vi "Test Read Speed.vi"(8 "error in (no error)":errorcluster, 11 "Path":path) -> (0 "error out":errorcluster, 2 "Read Times":T1)   [LabVIEW 2016]
uses:
  Data/Typedefs/Dictionary--cluster.ctl
  Data/Data.lvclass
  <vilib>/Utility/Data Type/NI_Data Type.lvlib
panel:
  out "Data (Dictionary)":T2[](array[typedef])=[{"key"="time", "value"=variant(dbl[] array[87118 elements])}, {"key"="temp", "value"=variant(dbl[] array[87118 elements])}, {"key"="Bfield", "value"=variant(dbl[] array[87118 elements])}, {"key"="X0", "value"=variant(dbl[] array[87118 elements])}, {"key"="Y0", "value"=variant(dbl[] array[87118 elements])}, {"key"="X1", "value"=variant(dbl[] array[87118 elements])}, {"key"="Y1", "value"=variant(dbl[] array[87118 elements])}, {"key"="X2", "value"=variant(dbl[] array[87118 elements])}, {"key"="Y2", "value"=variant(dbl[] array[87118 elements])}, {"key"="X3", "value"=variant(dbl[] array[87118 elements])}, {"key"="Y3", "value"=variant(dbl[] array[87118 elements])}, {"key"="X4", "value"=variant(dbl[] array[87118 elements])}, {"key"="Y4", "value"=variant(dbl[] array[87118 elements])}, {"key"="X5", "value"=variant(dbl[] array[87118 elements])}, {"key"="Y5", "value"=variant(dbl[] array[87118 elements])}, {"key"="X6", "value"=variant(dbl[] array[87118 elements])}, {"key"="Y6", "value"=variant(dbl[] array[87118 elements])}, {"key"="X7", "value"=variant(dbl[] array[87118 elements])}, {"key"="Y7", "value"=variant(dbl[] array[87118 elements])}]
  out "State":string
  in  "OK":bool
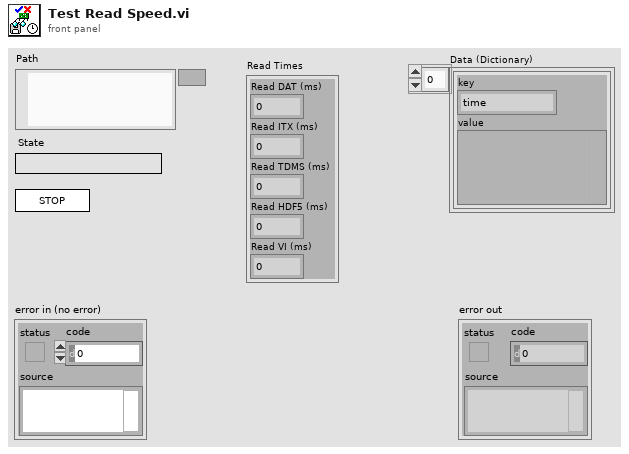
[diagram p1: front panel]
types:
  T1 = cluster{"Read DAT (ms)":u32, "Read ITX (ms)":u32, "Read TDMS (ms)":u32, "Read HDF5 (ms)":u32, "Read VI (ms)":u32}
  T2 = typedef "Data.lvclass/Dictionary--cluster.ctl" = cluster{"key":string, "value":variant}
  T3 = enum32{"Invalid", "Standard", "Closed", "Hidden", "Minimized", "Maximized"}
  T4 = enum32{"invalid app kind", "Development System", "Run Time System", "Student Edition", "Embedded LabVIEW", "Evaluation", "Custom"}
  T5 = cluster{"Core":cluster{"Current VI Reference":refnum<vi>, "Close Panel on Exit?":bool}, "Path":path, "Read Times":cluster{"Read DAT (ms)":u32, "Read ITX (ms)":u32, "Read TDMS (ms)":u32, "Read HDF5 (ms)":u32, "Read VI (ms)":u32}}
  T6 = cluster{"Current VI Reference":refnum<vi>, "Close Panel on Exit?":bool}
  T7 = typedef "NI_Data Type.lvlib/Data Type.ctl" = enum8{"Invalid Type", "Void", "I8", "I16", "I32", "I64", "U8", "U16", "U32", "U64", "Single Float", "Double Float", "Extended Float", "Single Complex", "Double Complex", "Extended Complex", "Enum U8", "Enum U16", "Enum U32", "Enum U64", "Single Float With Unit", "Double Float With Unit", "Extended Float With Unit", "Single Complex with Unit", "Double Complex with Unit", "Extended Complex with Unit", "Boolean", "String", "Path", "Picture", "Tag", "Array", "Cluster", "Variant", "LV Variant", "Waveform", "Timestamp", "Digital Waveform", "Digital Data", "ExpressData", "Refnum", "External Data", "VI", "Poly VI", "LabVIEW Class Instance", "Fixed Point"}
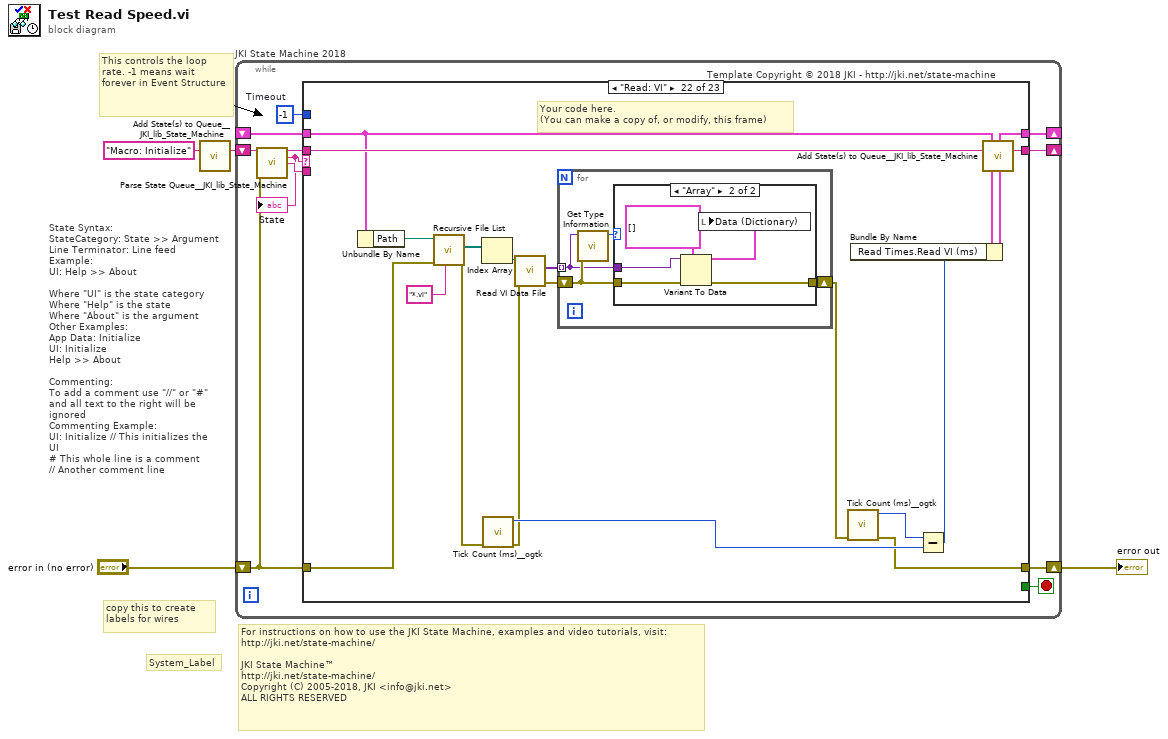
[diagram p0: block diagram]
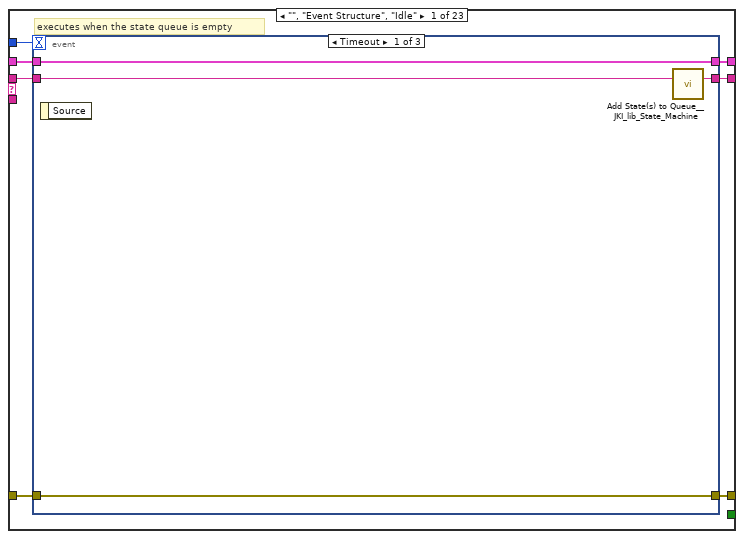
[diagram p2: hidden frame]
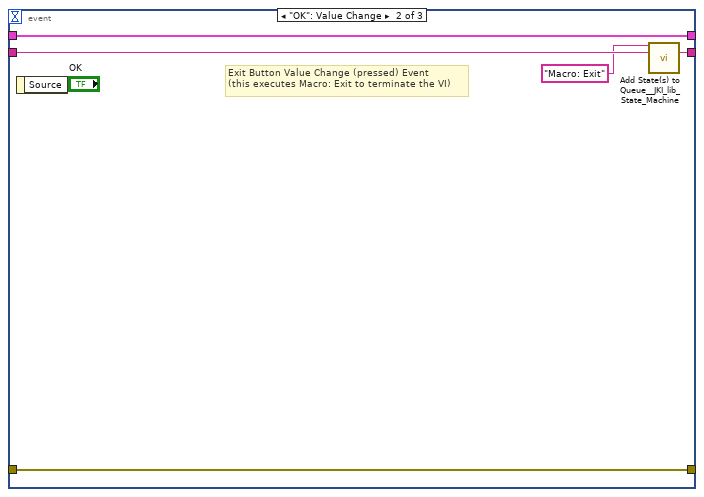
[diagram p3: hidden frame]
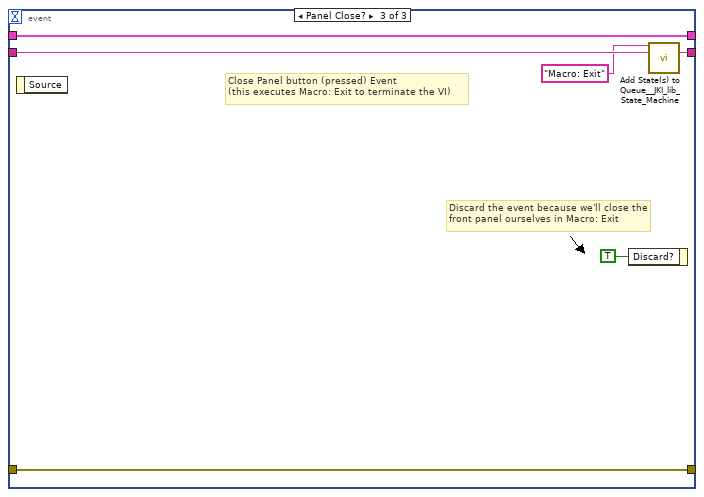
[diagram p4: hidden frame]
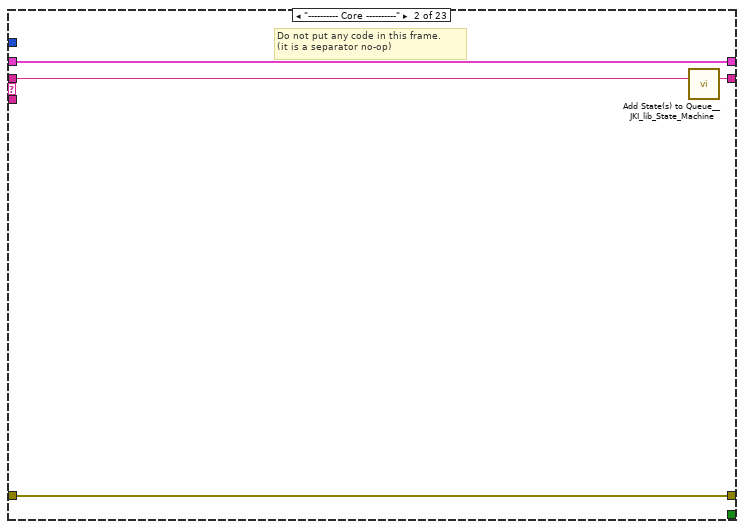
[diagram p5: hidden frame]
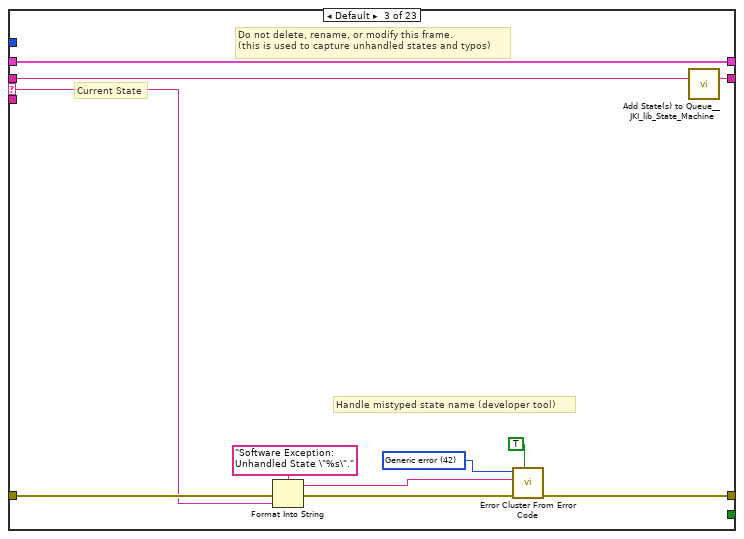
[diagram p6: hidden frame]
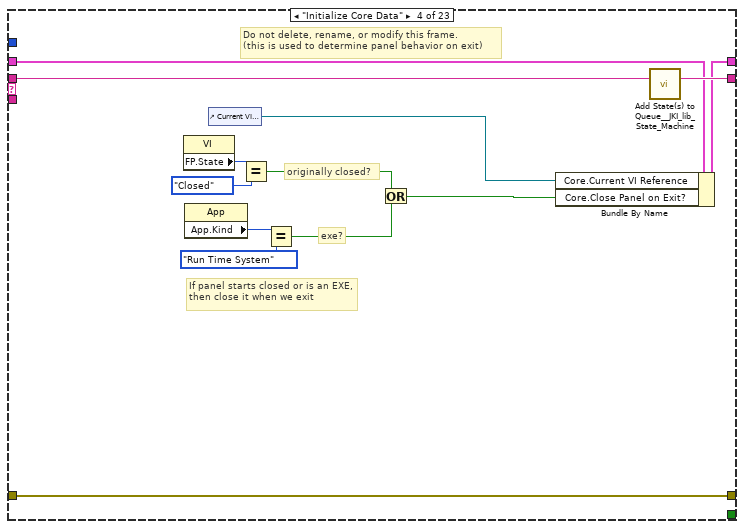
[diagram p7: hidden frame]
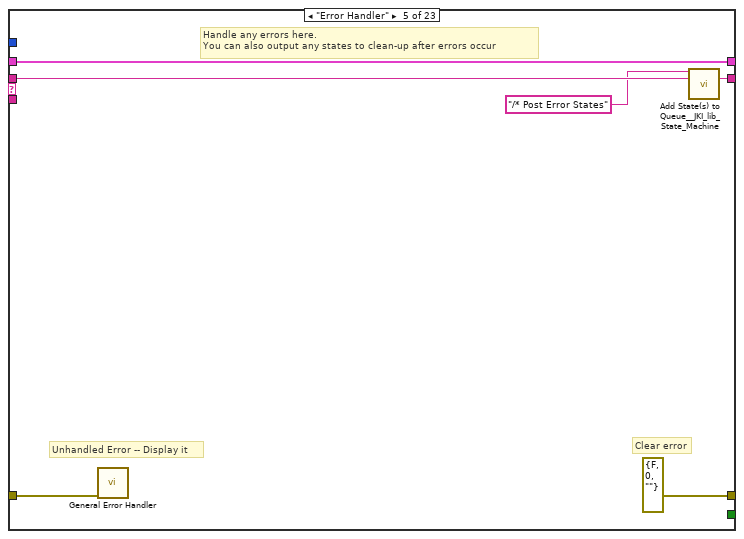
[diagram p8: hidden frame]
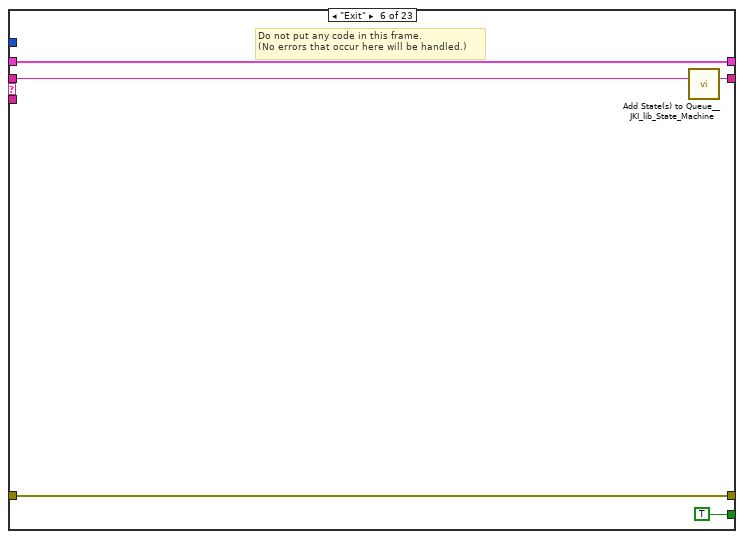
[diagram p9: hidden frame]
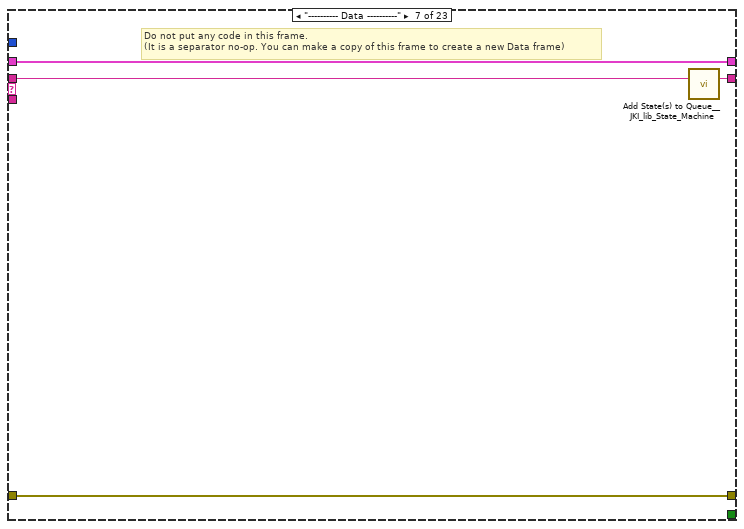
[diagram p10: hidden frame]
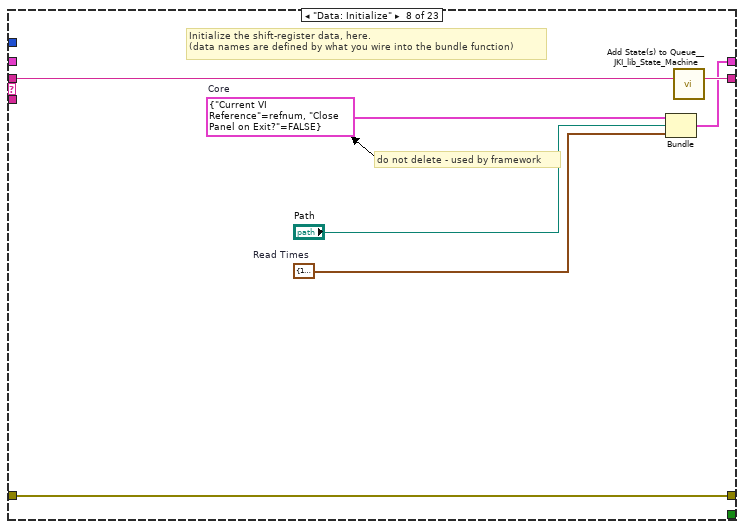
[diagram p11: hidden frame]
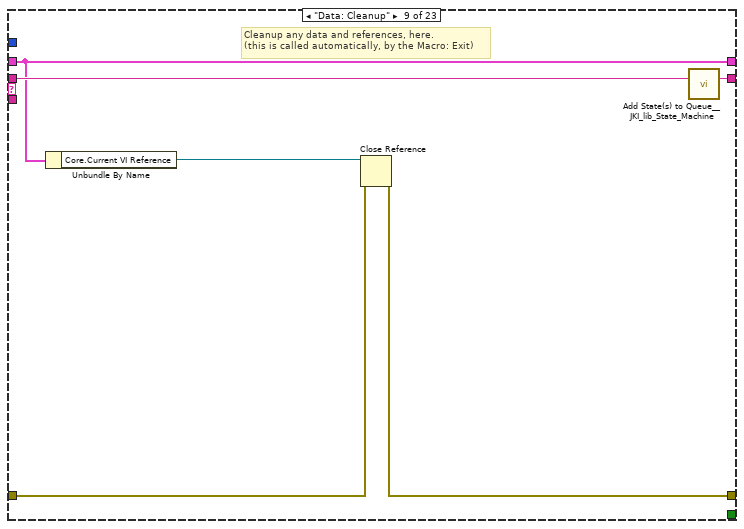
[diagram p12: hidden frame]
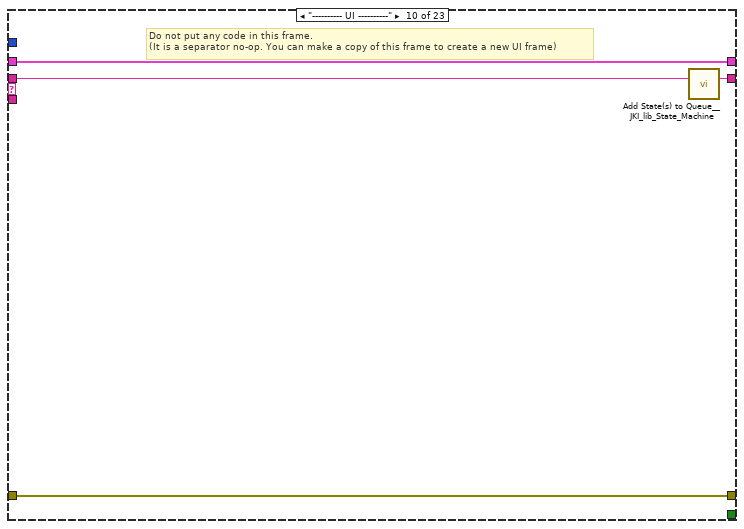
[diagram p13: hidden frame]
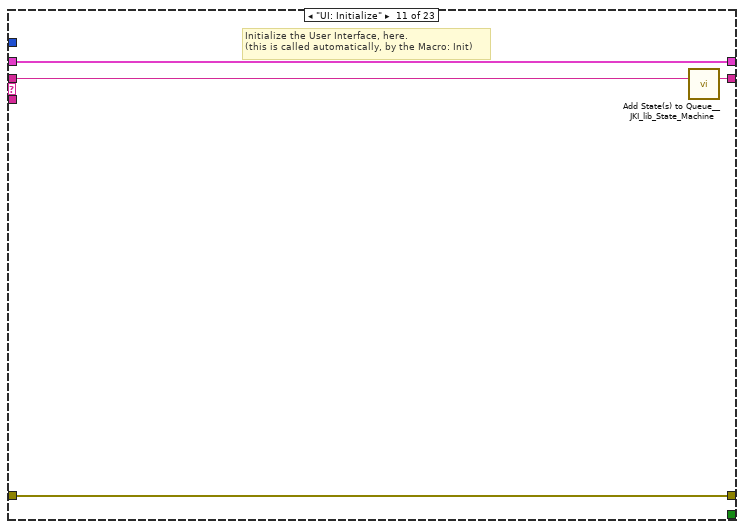
[diagram p14: hidden frame]
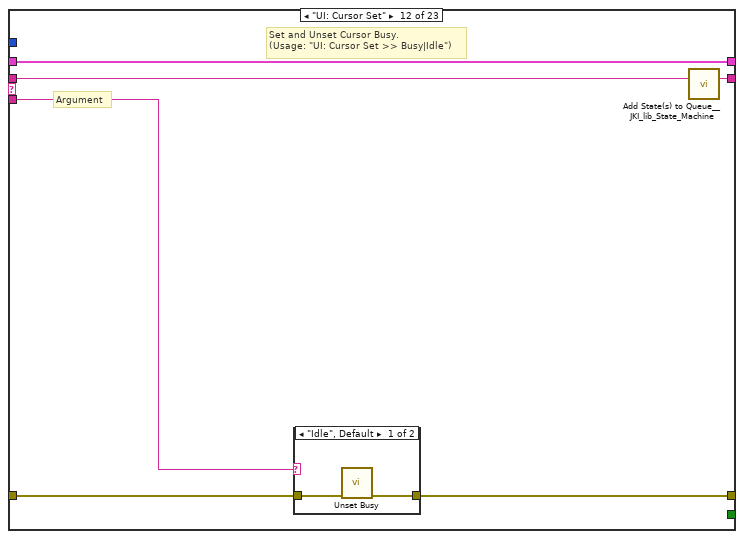
[diagram p15: hidden frame]
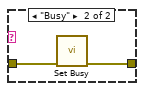
[diagram p16: hidden frame]
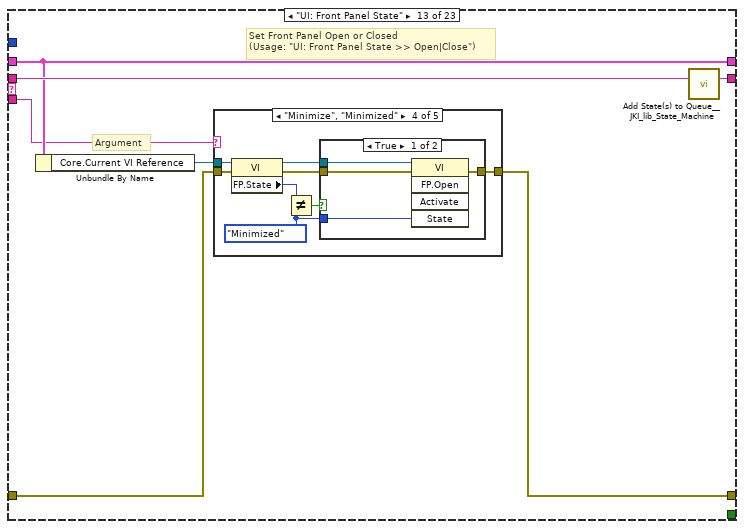
[diagram p17: hidden frame]
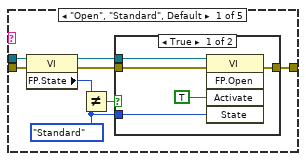
[diagram p18: hidden frame]
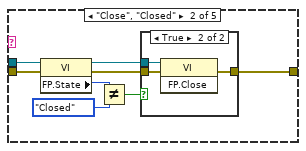
[diagram p20: hidden frame]
diagram:
  # "For instructions on how to use the JKI State Machine, examples and video tutorials, visit:\nhttp://jki.net/state-machine/\n\nJKI State Machine™\nhttp://jki.net/state-machine/\nCopyright (C) 2005-2018, JKI <info@jki.net>\nALL RIGHTS RESERVED"
  # "State Syntax:\nStateCategory: State >> Argument\nLine Terminator: Line feed\nExample:\nUI: Help >> About\n\nWhere \"UI\" is the state category\nWhere \"Help\" is the state\nWhere \"About\" is the argument\nOther Examples:\nApp Data: Initialize\nUI: Initialize\nHelp >> About\n\nCommenting:\nTo add a comment use \"//\" or \"#\" and all text to the right will be ignored\nCommenting Example:\nUI: Initialize // This initializes the UI\n# This whole line is a comment\n// Another comment line"
  # "copy this to create labels for wires"
  # "This controls the loop rate. -1 means wait forever in Event Structure"
  # "System_Label"
  n1 = call <vilib>:"Add State(s) to Queue__JKI_lib_State_Machine.vi"("State(s) in (\"\")"="Macro: Initialize") -> ("States Out"=w4:string)  [unwired: 14 in]
  n2 = while "JKI State Machine 2018" {
    shift-right: [w9] -> _
    shift-left: _ -> [w8]
    shift-right: [w12] -> w1
    shift-left: "error in (no error)" -> [w6]
    shift-right: [w11] -> _
    shift-left: w4 -> [w13]
    stop <- w10 stop-if-true
    w7 = -1  # Timeout
    # "Template Copyright © 2018 JKI - http://jki.net/state-machine"
    n3 = call <vilib>:"Parse State Queue__JKI_lib_State_Machine.vi"("State Queue"=w13, "Error In (no error)"=w6) -> ("Remaining States"=w15:string, "Current State"=w5:string, "Arguments"=w14:string)  [unwired: 11 in]
    "State" <- w5
    n4 = case shown="\"Read: VI\"" w5 {
      selector: w5 -> [_ _ w42 _ _ _ _ _ _ _ _ _ _ _ _ _ _ _ _ _ _ _ _]
      tunnel: w15 -> [w22 w41 w46 w65 w71 w76 w80 w87 w93 w97 w101 w107 w118 w187 w192 w197 w207 w211 w228 w245 w262 w280 w295]
      tunnel: w14 -> [_ _ _ _ _ _ _ _ _ _ _ w102 w112 _ _ _ _ _ _ _ _ _ _]
      tunnel: w8 -> [w20 w38 w44 w58 w68 w74 w77 _ w88 w94 w99 w105 w114 w184 w189 w194 w204 w208 w218 w234 w252 w264 w292]
      tunnel: [w19 w39 w48 w62 errorcluster {"status"=FALSE, "code"=0, "source"=""} ("error out") w73 w78 w84 w89 w95 w98 w103 w115 w185 w190 w195 w205 w209 w221 w239 w255 w273 w293] -> w12
      tunnel: w6 -> [w18 w39 w47 w62 w67 w73 w78 w84 w90 w95 w98 w104 w116 w185 w190 w195 w205 w209 w222 w240 w256 w274 w293]
      tunnel: [w21 w40 w45 w64 w70 w75 w79 w86 w92 w96 w100 w106 w117 w186 w191 w196 w206 w210 w227 w244 w261 w279 w294] -> w11
      tunnel: [_ _ _ _ _ TRUE _ _ _ _ _ _ _ _ _ _ _ _ _ _ _ _ _] -> w10
      tunnel: [w17 w38 w44 w63 w68 w74 w77 w85 w88 w94 w99 w105 w114 w184 w189 w194 w204 w208 w217 w233 w251 w263 w292] -> w9
      tunnel: w7 -> [w16 _ _ _ _ _ _ _ _ _ _ _ _ _ _ _ _ _ _ _ _ _ _]
      frame "", "Event Structure", "Idle" {
        # "executes when the state queue is empty"
        n5 = event shown="[0] Timeout" {
          selector: _ -> [_ _ _]
          dyn-events: _ -> [_ _ _]
          timeout: w16 -> [_ _ _]
          tunnel: w22 -> [w26 w31 w37]
          tunnel: [w25 w30 w36] -> w21
          tunnel: w20 -> [w23 w28 w34]
          tunnel: [w24 w29 w35] -> w19
          tunnel: w18 -> [w24 w29 w35]
          tunnel: [w23 w28 w34] -> w17
          event Timeout {
            n6 = event-data() -> ()  [unwired: 1 in, 1 out]
            n7 = call <vilib>:"Add State(s) to Queue__JKI_lib_State_Machine.vi"("State(s) in (\"\")"=w26) -> ("States Out"=w25:string)  [unwired: 14 in]
          }
          event "OK": Value Change {
            # "Exit Button Value Change (pressed) Event\n(this executes Macro: Exit to terminate the VI)"
            n8 = event-data() -> ()  [unwired: 1 in, 1 out]
            n9 = call <vilib>:"Add State(s) to Queue__JKI_lib_State_Machine.vi"("State(s) in Front (\"\")"="Macro: Exit", "State(s) in (\"\")"=w31) -> ("States Out"=w30:string)  [unwired: 13 in]
          }
          event Panel Close? {
            # "Discard the event because we'll close the front panel ourselves in Macro: Exit"
            # "Close Panel button (pressed) Event\n(this executes Macro: Exit to terminate the VI)"
            n10 = event-data() -> ()  [unwired: 1 in, 1 out]
            n11 = event-data("Discard?"=TRUE) -> ()  [unwired: 1 in, 1 out]
            n12 = call <vilib>:"Add State(s) to Queue__JKI_lib_State_Machine.vi"("State(s) in Front (\"\")"="Macro: Exit", "State(s) in (\"\")"=w37) -> ("States Out"=w36:string)  [unwired: 13 in]
          }
        }
      }
      frame "---------- Core ----------" {
        # "Do not put any code in this frame.\n(it is a separator no-op)"
        n13 = call <vilib>:"Add State(s) to Queue__JKI_lib_State_Machine.vi"("State(s) in (\"\")"=w41) -> ("States Out"=w40:string)  [unwired: 14 in]
      }
      frame Default {
        w51 = 42 items=["No error", "Argument error", "Memory is full", "Out of zone", "End of file", "File already open", "Generic file I/O error", "File not found", "File permission error", "Disk is full", "Duplicate path", "Too many files open", "System feature not enabled", "Resource file not found", "Cannot add resource", "Resource not found", "Image not found", "Image memory error", "Pen does not exist", "Config type invalid", "Config token not found", "Config parse error", "Config memory error", "Bad external code format", "Bad external code offset", "External code not present", "Null window", "Destroy window error", "Null menu", "Print aborted", "Bad print record", "Print driver error", "Windows error during printing", "Memory error during printing", "Print dialog error", "Generic print error", "Invalid device refnum", "Device not found", "Device parameter error", "Device unit error", "Cannot open device", "Device call aborted", "Generic error", "Cancelled by user", "Object ID too low", "Object ID too high", "Object not in heap", "Unknown heap", "Unknown object (invalid DefProc)", "Unknown object (DefProc not in table)", "Message out of range", "Invalid (null) method", "Unknown message", "Manager call not supported", "Bad address", "Network operation in progress", "Network operation timed out", "Connection is busy", "Network attribute not supported", "Network error", "Address in use", "System out of memory", "Connection aborted", "Connection refused", "Not connected", "Already connected", "Connection closed", "Initialization error (interapplication manager)", "Bad occurrence", "Wait on unbound occurrence handler", "Occurrence queue overflow", "Datalog type conflict", "Unused", "Unrecognized type (interapplication manager)", "Memory corrupt", "Failed to make temporary DLL", "Old CIN version", "Drag socket not found", "Failed to load drop-object", "Failed to register OLE object", "Failed to release OLE object", "Format specifier type mismatch", "Unknown format specifier", "Too few format specifiers", "Too many format specifiers", "Scan failed", "Newer CIN version", "Error converting to variant", "Runtime menu error", "Password tampered", "Variant attribute not found", "Incompatible variant data type", "Event data is not available", "Event Store is not present", "Occurrence is not found", "Event Queue is not created", "Event info is not available", "Refnum passed is NULL", "Error retrieving Class GUID", "Error retrieving CoClass GUID", "Error retrieving TypeLib GUID.", "Bad built application magic bytes.", "Specific driver is different from the specific driver associated with the Logical Name.", "There is no session opened to the class driver.", "Max Error", "MAX - Error with config objects", "MAX - Error loading configuration", "MAX - Group not supported"]
        # "Current State"
        # "Do not delete, rename, or modify this frame.\n(this is used to capture unhandled states and typos)"
        # "Handle mistyped state name (developer tool)"
        n14 = Format Into String(format string="Software Exception: Unhandled State \"%s\"." ("message"), error in=w47, w42) -> (resulting string=w50:string, error out=w49:errorcluster)  [unwired: 1 in]
        n15 = call <vilib>:"Error Cluster From Error Code.vi"("show call chain? (False)"=TRUE, "error in (no error)"=w49, "error message (\"\")"=w50, "error code (0)"=w51) -> ("error out"=w48:errorcluster)  [unwired: 5 in]
        n16 = call <vilib>:"Add State(s) to Queue__JKI_lib_State_Machine.vi"("State(s) in (\"\")"=w46) -> ("States Out"=w45:string)  [unwired: 14 in]
      }
      frame "Initialize Core Data" {
        # "Do not delete, rename, or modify this frame.\n(this is used to determine panel behavior on exit)"
        # "originally closed?"
        # "exe?"
        # "If panel starts closed or is an EXE, then close it when we exit"
        n17 = property class="VI"() -> ("FP.State"=w55:T3)  [unwired: 2 in, 2 out]
        n18 = property class="App"() -> ("App.Kind"=w61:T4)  [unwired: 2 in, 2 out]
        n19 = control-ref of="Current VI Reference"() -> (w56:refnum<vi>)
        n20 = Equal?(x=w55, y=T3."Closed" ("Front Panel Window:State")) -> (x = y?=w53:bool)
        n21 = Equal?(x=w61, y=T4."Run Time System" ("Application:Kind")) -> (x = y?=w59:bool)
        n22 = Or(x=w53, y=w59) -> (x .or. y?=w57:bool)
        n23 = Bundle By Name(cluster=w58, "Core.Current VI Reference"=w56, "Core.Close Panel on Exit?"=w57) -> (w63:T5)
        n24 = call <vilib>:"Add State(s) to Queue__JKI_lib_State_Machine.vi"("State(s) in (\"\")"=w65) -> ("States Out"=w64:string)  [unwired: 14 in]
      }
      frame "Error Handler" {
        # "Unhandled Error -- Display it"
        # "Handle any errors here.\nYou can also output any states to clean-up after errors occur"
        # "Clear error"
        n25 = call <vilib>:"General Error Handler.vi"("error in (no error)"=w67) -> ()  [unwired: 10 in, 5 out]
        n26 = call <vilib>:"Add State(s) to Queue__JKI_lib_State_Machine.vi"("State(s) in Front (\"\")"="/* Post Error States", "State(s) in (\"\")"=w71) -> ("States Out"=w70:string)  [unwired: 13 in]
      }
      frame "Exit" {
        # "Do not put any code in this frame.\n(No errors that occur here will be handled.)"
        n27 = call <vilib>:"Add State(s) to Queue__JKI_lib_State_Machine.vi"("State(s) in (\"\")"=w76) -> ("States Out"=w75:string)  [unwired: 14 in]
      }
      frame "---------- Data ----------" {
        # "Do not put any code in this frame.\n(It is a separator no-op. You can make a copy of this frame to create a new Data frame)"
        n28 = call <vilib>:"Add State(s) to Queue__JKI_lib_State_Machine.vi"("State(s) in (\"\")"=w80) -> ("States Out"=w79:string)  [unwired: 14 in]
      }
      frame "Data: Initialize" {
        w81 = T1 {"Read DAT (ms)"=1332, "Read ITX (ms)"=1743, "Read TDMS (ms)"=84, "Read HDF5 (ms)"=43, "Read VI (ms)"=279}  # Read Times
        w83 = T6 {"Current VI Reference"=refnum, "Close Panel on Exit?"=FALSE}  # Core
        # "do not delete - used by framework"
        # "Initialize the shift-register data, here.\n(data names are defined by what you wire into the bundle function)"
        n29 = Bundle("Core"=w83, "Path"="Path", "Read Times"=w81) -> (w85:T5)  [unwired: 1 in]
        n30 = call <vilib>:"Add State(s) to Queue__JKI_lib_State_Machine.vi"("State(s) in (\"\")"=w87) -> ("States Out"=w86:string)  [unwired: 14 in]
      }
      frame "Data: Cleanup" {
        # "Cleanup any data and references, here.\n(this is called automatically, by the Macro: Exit)"
        n31 = Unbundle By Name(w88) -> ("Core.Current VI Reference"=w91:refnum<vi>)
        n32 = Close Reference(reference=w91, error in (no error)=w90) -> (error out=w89:errorcluster)
        n33 = call <vilib>:"Add State(s) to Queue__JKI_lib_State_Machine.vi"("State(s) in (\"\")"=w93) -> ("States Out"=w92:string)  [unwired: 14 in]
      }
      frame "---------- UI ----------" {
        # "Do not put any code in this frame.\n(It is a separator no-op. You can make a copy of this frame to create a new UI frame)"
        n34 = call <vilib>:"Add State(s) to Queue__JKI_lib_State_Machine.vi"("State(s) in (\"\")"=w97) -> ("States Out"=w96:string)  [unwired: 14 in]
      }
      frame "UI: Initialize" {
        # "Initialize the User Interface, here.\n(this is called automatically, by the Macro: Init)"
        n35 = call <vilib>:"Add State(s) to Queue__JKI_lib_State_Machine.vi"("State(s) in (\"\")"=w101) -> ("States Out"=w100:string)  [unwired: 14 in]
      }
      frame "UI: Cursor Set" {
        # "Argument"
        # "Set and Unset Cursor Busy.\n(Usage: \"UI: Cursor Set >> Busy|Idle\")"
        n36 = case shown="\"Idle\", Default" w102 {
          tunnel: w104 -> [w109 w111]
          tunnel: [w108 w110] -> w103
          frame "Idle", Default {
            n37 = call <vilib>:"Unset Busy.vi"("error in (no error)"=w109) -> ("error out"=w108:errorcluster)  [unwired: 10 in]
          }
          frame "Busy" {
            n38 = call <vilib>:"Set Busy.vi"("error in (no error)"=w111) -> ("error out"=w110:errorcluster)  [unwired: 9 in, 1 out]
          }
        }
        n39 = call <vilib>:"Add State(s) to Queue__JKI_lib_State_Machine.vi"("State(s) in (\"\")"=w107) -> ("States Out"=w106:string)  [unwired: 14 in]
      }
      frame "UI: Front Panel State" {
        # "Argument"
        # "Set Front Panel Open or Closed\n(Usage: \"UI: Front Panel State >> Open|Close\")"
        n40 = Unbundle By Name(w114) -> ("Core.Current VI Reference"=w113:refnum<vi>)
        n41 = case shown="\"Minimize\", \"Minimized\"" w112 {
          tunnel: w116 -> [w124 w139 w150 w163 w176]
          tunnel: [w126 w140 w152 w165 w178] -> w115
          tunnel: w113 -> [w125 w137 w151 w164 w177]
          frame "Open", "Standard", Default {
            w119 = T3."Standard" ("State")
            n42 = property class="VI"(reference=w125, error in=w124) -> (reference out=w122:refnum<vi>, error out=w123:errorcluster, "FP.State"=w121:T3)
            n43 = Not Equal?(x=w121, y=w119) -> (x != y?=w120:bool)
            n44 = case shown="True" w120 {
              tunnel: [w130 w132] -> w126
              tunnel: w123 -> [w129 w132]
              tunnel: w122 -> [w128 _]
              tunnel: w119 -> [w127 _]
              frame True {
                n45 = invoke class="VI" method="FP.Open"(reference=w128, error in=w129, "Activate"=TRUE, "State"=w127) -> (error out=w130:errorcluster)  [unwired: 1 in, 4 out]
              }
              frame False {
              }
            }
          }
          frame "Close", "Closed" {
            n46 = property class="VI"(reference=w137, error in=w139) -> (reference out=w136:refnum<vi>, error out=w138:errorcluster, "FP.State"=w134:T3)
            n47 = Not Equal?(x=w134, y=T3."Closed" ("Front Panel Window:State")) -> (x != y?=w133:bool)
            n48 = case shown="True" w133 {
              tunnel: [w141 w144] -> w140
              tunnel: w138 -> [w141 w143]
              tunnel: w136 -> [_ w142]
              frame False {
              }
              frame True {
                n49 = invoke class="VI" method="FP.Close"(reference=w142, error in=w143) -> (error out=w144:errorcluster)  [unwired: 1 in, 2 out]
              }
            }
          }
          frame "Hidden", "Hide" {
            w145 = T3."Hidden" ("State")
            n50 = property class="VI"(reference=w151, error in=w150) -> (reference out=w148:refnum<vi>, error out=w149:errorcluster, "FP.State"=w147:T3)
            n51 = Not Equal?(x=w147, y=w145) -> (x != y?=w146:bool)
            n52 = case shown="True" w146 {
              tunnel: [w156 w157] -> w152
              tunnel: w149 -> [w155 w157]
              tunnel: w148 -> [w154 _]
              tunnel: w145 -> [w153 _]
              frame True {
                n53 = invoke class="VI" method="FP.Open"(reference=w154, error in=w155, "State"=w153) -> (error out=w156:errorcluster)  [unwired: 2 in, 4 out]
              }
              frame False {
              }
            }
          }
          frame "Minimize", "Minimized" {
            w158 = T3."Minimized" ("State")
            n54 = property class="VI"(reference=w164, error in=w163) -> (reference out=w161:refnum<vi>, error out=w162:errorcluster, "FP.State"=w160:T3)
            n55 = Not Equal?(x=w160, y=w158) -> (x != y?=w159:bool)
            n56 = case shown="True" w159 {
              tunnel: [w169 w170] -> w165
              tunnel: w162 -> [w168 w170]
              tunnel: w161 -> [w167 _]
              tunnel: w158 -> [w166 _]
              frame True {
                n57 = invoke class="VI" method="FP.Open"(reference=w167, error in=w168, "State"=w166) -> (error out=w169:errorcluster)  [unwired: 2 in, 4 out]
              }
              frame False {
              }
            }
          }
          frame "Maximize", "Maximized" {
            w171 = T3."Maximized" ("State")
            n58 = property class="VI"(reference=w177, error in=w176) -> (reference out=w174:refnum<vi>, error out=w175:errorcluster, "FP.State"=w173:T3)
            n59 = Not Equal?(x=w173, y=w171) -> (x != y?=w172:bool)
            n60 = case shown="True" w172 {
              tunnel: [w182 w183] -> w178
              tunnel: w175 -> [w181 w183]
              tunnel: w174 -> [w180 _]
              tunnel: w171 -> [w179 _]
              frame True {
                n61 = invoke class="VI" method="FP.Open"(reference=w180, error in=w181, "State"=w179) -> (error out=w182:errorcluster)  [unwired: 2 in, 4 out]
              }
              frame False {
              }
            }
          }
        }
        n62 = call <vilib>:"Add State(s) to Queue__JKI_lib_State_Machine.vi"("State(s) in (\"\")"=w118) -> ("States Out"=w117:string)  [unwired: 14 in]
      }
      frame "---------- Macro ----------" {
        # "Do not put any code in this frame.\n(It is a separator no-op. You can make a copy of this frame to create a new Macro frame)"
        n63 = call <vilib>:"Add State(s) to Queue__JKI_lib_State_Machine.vi"("State(s) in (\"\")"=w187) -> ("States Out"=w186:string)  [unwired: 14 in]
      }
      frame "Macro: Initialize" {
        w188 = "Data: Initialize\nInitialize Core Data\nUI: Initialize\nUI: Front Panel State >> Open\nMacro: Read"  # Data: Initialize Initialize Core Data UI: Initialize UI: Front Panel State >> Open Macro: Read
        # "Initialization Macro\n(This is called once, when the VI starts)"
        n64 = call <vilib>:"Add State(s) to Queue__JKI_lib_State_Machine.vi"("State(s) in Front (\"\")"=w188, "State(s) in (\"\")"=w192) -> ("States Out"=w191:string)  [unwired: 13 in]
      }
      frame "Macro: Read" {
        # "Do not put any code in this frame.\n(It is a separator no-op. You can make a copy of this frame to create a new Macro frame)"
        n65 = call <vilib>:"Add State(s) to Queue__JKI_lib_State_Machine.vi"("State(s) in Front (\"\")"="Read: DAT\nRead: ITX\nRead: TDMS\n//Read: VI\nRead: Update\nMacro: Exit", "State(s) in (\"\")"=w197) -> ("States Out"=w196:string)  [unwired: 13 in]
      }
      frame "Macro: Exit" {
        # "Exit Macro\n(This is called once, when the VI exits)"
        n66 = Unbundle By Name(w204) -> ("Core.Close Panel on Exit?"=w203:bool)
        n67 = Select(t="UI: Front Panel State >> Close", s=w203, f="") -> (s? t:f=w200:string)
        n68 = call <vilib>:"Add State(s) to Queue__JKI_lib_State_Machine.vi"("State(s) in (\"\")"=w200, "State(s) at Back (\"\")"="Data: Cleanup\nExit") -> ("States Out"=w198:string)  [unwired: 13 in]
        n69 = call <vilib>:"Add State(s) to Queue__JKI_lib_State_Machine.vi"("State(s) in Front (\"\")"=w198, "State(s) in (\"\")"=w207) -> ("States Out"=w206:string)  [unwired: 13 in]
      }
      frame "---------- Read ----------" {
        # "Template Separator\n(You can make a copy of, or modify, this frame)"
        n70 = call <vilib>:"Add State(s) to Queue__JKI_lib_State_Machine.vi"("State(s) in (\"\")"=w211) -> ("States Out"=w210:string)  [unwired: 14 in]
      }
      frame "Read: DAT" {
        # "Your code here.\n(You can make a copy of, or modify, this frame)"
        n71 = Unbundle By Name(w218) -> ("Path"=w220:path)
        n72 = call <vilib>:"Recursive File List.vi"("pattern"="*.dat", "error in (no error)"=w222, "Folder Path"=w220) -> ("error out"=w226:errorcluster, "All Files in Dir"=w223:path[])  [unwired: 4 in, 3 out]
        n73 = call <userlib>:"Tick Count (ms)__ogtk.vi"("error in (no error)"=w226) -> ("error out"=w214:errorcluster, "millisecond timer value"=w225:u32)  [unwired: 9 in]
        n74 = Index Array(array=w223) -> (element=w215:path)  [unwired: 1 in]
        n75 = call "Data Read.vi"("error in (no error)"=w214, "path"=w215) -> ("error out"=w213:errorcluster, "Data (Dictionary)"=w212:T2[])  [unwired: 6 in, 2 out]
        n76 = local write "Data (Dictionary)"(w212) -> ()
        n77 = call <userlib>:"Tick Count (ms)__ogtk.vi"("error in (no error)"=w213) -> ("error out"=w221:errorcluster, "millisecond timer value"=w224:u32)  [unwired: 9 in]
        n78 = Subtract(x=w224, y=w225) -> (x-y=w216:u32)
        n79 = Bundle By Name(cluster=w218, "Read Times.Read DAT (ms)"=w216) -> (w217:T5)
        n80 = call <vilib>:"Add State(s) to Queue__JKI_lib_State_Machine.vi"("State(s) in (\"\")"=w228) -> ("States Out"=w227:string)  [unwired: 14 in]
      }
      frame "Read: ITX" {
        # "Your code here.\n(You can make a copy of, or modify, this frame)"
        n81 = Unbundle By Name(w234) -> ("Path"=w238:path)
        n82 = call <vilib>:"Recursive File List.vi"("pattern"="*.itx", "error in (no error)"=w240, "Folder Path"=w238) -> ("error out"=w243:errorcluster, "All Files in Dir"=w241:path[])  [unwired: 4 in, 3 out]
        n83 = call <userlib>:"Tick Count (ms)__ogtk.vi"("error in (no error)"=w243) -> ("error out"=w230:errorcluster, "millisecond timer value"=w236:u32)  [unwired: 9 in]
        n84 = Index Array(array=w241) -> (element=w232:path)  [unwired: 1 in]
        n85 = call "Data Read.vi"("error in (no error)"=w230, "path"=w232) -> ("error out"=w229:errorcluster, "Data (Dictionary)"=w231:T2[])  [unwired: 6 in, 2 out]
        n86 = local write "Data (Dictionary)"(w231) -> ()
        n87 = call <userlib>:"Tick Count (ms)__ogtk.vi"("error in (no error)"=w229) -> ("error out"=w239:errorcluster, "millisecond timer value"=w242:u32)  [unwired: 9 in]
        n88 = Subtract(x=w242, y=w236) -> (x-y=w235:u32)
        n89 = Bundle By Name(cluster=w234, "Read Times.Read ITX (ms)"=w235) -> (w233:T5)
        n90 = call <vilib>:"Add State(s) to Queue__JKI_lib_State_Machine.vi"("State(s) in (\"\")"=w245) -> ("States Out"=w244:string)  [unwired: 14 in]
      }
      frame "Read: TDMS" {
        # "Your code here.\n(You can make a copy of, or modify, this frame)"
        n91 = Unbundle By Name(w252) -> ("Path"=w254:path)
        n92 = call <vilib>:"Recursive File List.vi"("pattern"="*.tdms", "error in (no error)"=w256, "Folder Path"=w254) -> ("error out"=w260:errorcluster, "All Files in Dir"=w257:path[])  [unwired: 4 in, 3 out]
        n93 = call <userlib>:"Tick Count (ms)__ogtk.vi"("error in (no error)"=w260) -> ("error out"=w248:errorcluster, "millisecond timer value"=w259:u32)  [unwired: 9 in]
        n94 = Index Array(array=w257) -> (element=w249:path)  [unwired: 1 in]
        n95 = call "Data Read.vi"("error in (no error)"=w248, "path"=w249) -> ("error out"=w247:errorcluster, "Data (Dictionary)"=→"Data (Dictionary)":T2[])  [unwired: 6 in, 2 out]
        n96 = call <userlib>:"Tick Count (ms)__ogtk.vi"("error in (no error)"=w247) -> ("error out"=w255:errorcluster, "millisecond timer value"=w258:u32)  [unwired: 9 in]
        n97 = Subtract(x=w258, y=w259) -> (x-y=w250:u32)
        n98 = Bundle By Name(cluster=w252, "Read Times.Read TDMS (ms)"=w250) -> (w251:T5)
        n99 = call <vilib>:"Add State(s) to Queue__JKI_lib_State_Machine.vi"("State(s) in (\"\")"=w262) -> ("States Out"=w261:string)  [unwired: 14 in]
      }
      frame "Read: VI" {
        # "Your code here.\n(You can make a copy of, or modify, this frame)"
        n100 = Unbundle By Name(w264) -> ("Path"=w272:path)
        n101 = call <vilib>:"Recursive File List.vi"("pattern"="*.vi", "error in (no error)"=w274, "Folder Path"=w272) -> ("error out"=w278:errorcluster, "All Files in Dir"=w275:path[])  [unwired: 4 in, 3 out]
        n102 = Index Array(array=w275) -> (element=w269:path)  [unwired: 1 in]
        n103 = call <userlib>:"Tick Count (ms)__ogtk.vi"("error in (no error)"=w278) -> ("error out"=w270:errorcluster, "millisecond timer value"=w277:u32)  [unwired: 9 in]
        n104 = call "Read VI Data File.vi"("error in"=w270, "Path"=w269) -> ("error out"=w267:errorcluster, "Data"=w268:variant[])  [unwired: 7 in, 1 out]
        n105 = for {
          tunnel: w268 -> [w281] mode=indexing
          shift-right: [w284] -> w266
          shift-left: w267 -> [w283]
          n106 = call <vilib>:"Get Type Information.vi"("error in (no error)"=w283, "Variant"=w281) -> ("Type"=w282:T7)  [unwired: 5 in, 4 out]
          n107 = case shown="\"Array\"" w282 {
            tunnel: w281 -> [_ w290]
            tunnel: w283 -> [w285 w288]
            tunnel: [w285 w287] -> w284
            frame "Invalid Type", Default {
            }
            frame "Array" {
              n108 = Variant To Data(error in=w288, type=T2[] [] ("Data (Dictionary)"), Variant=w290) -> (data=w286:T2[], error out=w287:errorcluster)
              n109 = local write "Data (Dictionary)"(w286) -> ()
            }
          }
        }
        n110 = call <userlib>:"Tick Count (ms)__ogtk.vi"("error in (no error)"=w266) -> ("error out"=w273:errorcluster, "millisecond timer value"=w276:u32)  [unwired: 9 in]
        n111 = Subtract(x=w276, y=w277) -> (x-y=w265:u32)
        n112 = Bundle By Name(cluster=w264, "Read Times.Read VI (ms)"=w265) -> (w263:T5)
        n113 = call <vilib>:"Add State(s) to Queue__JKI_lib_State_Machine.vi"("State(s) in (\"\")"=w280) -> ("States Out"=w279:string)  [unwired: 14 in]
      }
      frame "Read: Update" {
        # "Template Separator\n(You can make a copy of, or modify, this frame)"
        n114 = Unbundle By Name(w292) -> ("Read Times"=→"Read Times":T1)
        n115 = call <vilib>:"Add State(s) to Queue__JKI_lib_State_Machine.vi"("State(s) in (\"\")"=w295) -> ("States Out"=w294:string)  [unwired: 14 in]
      }
    }
  }
  "error out" <- w1
